vi "cRIO_8maze_controls_exo_wheelstart.vi"() -> ()   [LabVIEW 2019]
uses:
  <vilib>/Platform/TimedLoop/XDataNode/timing_clust.ctl
  <vilib>/Platform/TimedLoop/XDataNode/nitl_modes.ctl
  <vilib>/Platform/TimedLoop/XDataNode/wakeup.ctl
  Global 1.vi
  <vilib>/addons/control/pid/pid.llb/PID (DBL Array).vi
  <vilib>/imath/engines/lvmath2/RunTimeEngine/BuiltInFunctions/inv/NIMS_inv(GM).vi
  <instcachedir>/0/NIMS_inv(GM)_A6DF8FE880224208AACFE4CF9F659502.lvgen/NIMS_inv(GM)_A6DF8FE880224208AACFE4CF9F659502_000.vi
  <vilib>/imath/engines/lvmath2/RunTimeEngine/ArithmeticOperatorToken/NIMS_ArithmeticOperator_multmx(M,CV).vi
  <instcachedir>/0/NIMS_ArithmeticOperator_multmx(M,CV)_1D61EED49E1847F3B05DBB8EDD2FBF8F.lvgen/NIMS_ArithmeticOperator_multmx(M,CV)_1D61EED49E1847F3B05DBB8EDD2FBF8F_000.vi
  <vilib>/imath/engines/lvmath2/RunTimeEngine/ErrorHandling/NIMS_Create Error From Enums.vi
  <vilib>/imath/engines/lvmath2/RunTimeEngine/IndexRead/NIMS M(R2,S).vi
  <instcachedir>/0/NIMS M(R2,S)_56813DCFDD5A484292D2195AF15D2BF5.lvgen/NIMS M(R2,S)_56813DCFDD5A484292D2195AF15D2BF5_000.vi
  <vilib>/imathl/engines/lvmath/Functions/Error Handling/Create Error.vi
  <vilib>/imath/engines/lvmath2/RunTimeEngine/IndexRead/NIMS M(S,S).vi
  <instcachedir>/0/NIMS M(S,S)_AC51E74150A542F7991B9634C66F3096.lvgen/NIMS M(S,S)_AC51E74150A542F7991B9634C66F3096_000.vi
  <vilib>/imath/engines/lvmath2/RunTimeEngine/NodeEndStatement/NIMS_NodeEndStatement_Output.vi
  <instcachedir>/0/NIMS_NodeEndStatement_Output_53EC0D466D134D7ABD903AC30B43404B.lvgen/NIMS_NodeEndStatement_Output_53EC0D466D134D7ABD903AC30B43404B_001.vi
  <instcachedir>/0/NIMS_NodeEndStatement_Output_53EC0D466D134D7ABD903AC30B43404B.lvgen/NIMS_NodeEndStatement_Output_53EC0D466D134D7ABD903AC30B43404B_005.vi
  <vilib>/imath/engines/lvmath2/RunTimeEngine/ErrorHandling/NIMS_Finalize Error.vi
  <vilib>/platform/TimedLoop/XDataNode/XDataNode.xnode
  <vilib>/addons/control/pid/NI_PID_pid.lvlib
  <vilib>/Platform/TimedLoop/XDataNode/XDNodeRunTimeDep.lvlib
panel:
  in  "Reset sliders":bool=TRUE
  in  "MDServoPWM_R":dbl[](array[numeric])=[5.3, 8.5]
  in  "MDServoPWM_L":dbl[](array[numeric])=[4.6, 8.4]
  in  "Mouse off":bool
  in  "PWMset2":dbl[](array[numeric])=[8.1, 5.3, 8.5]
  in  "PWMset1":dbl[](array[numeric])=[3.4, 4.6, 8.2]
  in  "PWM positions":dbl[](array[numeric])=[8.7, 4.0, 4.4, 8.6]
  in  "PWM rate":dbl[](array[numeric])=[0.1, 0.1, 0.1, 0.1]
  out "appended array":bool[](array[boolean])
  in  "LED_L":bool
  in  "LED_R":bool
  in  "MD_L":bool
  in  "MD_R":bool
  out "Left":bool=TRUE
  in  "AIR":bool
  in  "Sound":bool
  out "Right":bool=TRUE
  in  "MD time (ms)":i32=3000
  in  "Loop seq.":dbl
  in  "Initialize":bool=TRUE
  in  "No Milk":bool
  out "All BBL":bool
  out "BB3_L":bool
  out "BB2_L":bool
  out "BB1_R":bool
  out "All BBR":bool
  out "BB3_R":bool
  out "BB2_R":bool
  out "BB1_L":bool
  out "Seq update":i32
  in  "Make sound":bool
  in  "Air puff time":u32=1000
  out "Direction array":bool[](array[boolean])=[TRUE, FALSE, FALSE, TRUE, FALSE, TRUE, TRUE, FALSE, TRUE, FALSE, FALSE, TRUE, FALSE, TRUE, FALSE, FALSE, TRUE, FALSE, TRUE, TRUE, FALSE, TRUE, FALSE, FALSE, TRUE, FALSE, TRUE, TRUE, FALSE, TRUE, FALSE, FALSE, TRUE, FALSE, TRUE, TRUE, FALSE, TRUE, FALSE, FALSE, TRUE, FALSE, TRUE, TRUE, FALSE, TRUE, FALSE, FALSE, TRUE]
  in  "manual homing stop":bool
  out "Homed":bool[](array[boolean])
  out "Hall voltages":dbl[](array[numeric])
  in  "Joint offset":dbl[](array[numeric])
  in  "Target HallV":dbl[](array[numeric])
  out "loop":i32
  in  "RETURN TO HOME \nPOSITION AND STOP":bool
  in  "lower limit":dbl[](array[numeric])=[-0.3, -0.36, -0.782, -6000.0]
  in  "upper limit":dbl[](array[numeric])=[0.3, 0.36, -0.65, 6000.0]
  in  "Yaw":dbl(slide) scale=0.0..3.142
  in  "Z":dbl(slide)=-0.7034810126582278 scale=-0.1..0.1
  in  "Y":dbl(slide) scale=-0.3..0.15
  in  "X":dbl(slide) scale=-0.15..0.15
  out "target position":dbl[](array[numeric])
  in  "Output range (PWM)":cluster{"output high":dbl, "output low":dbl}[](array[cluster])=[{"output high"=100.0, "output low"=-100.0}] {"output low" format="%.2f"; "output high" format="%.2f"}
  in  "Admittance PID gains":T1(array[cluster])=[{"proportional gain (Kc)"=1.0, "integral time (Ti, min)"=0.01, "derivative time (Td, min)"=0.0}] {"derivative time (Td, min)" format="%.3f"; "integral time (Ti, min)" format="%.3f"; "proportional gain (Kc)" format="%.3f"}
  in  "goniometer PWM\n offset":dbl=50.0
  in  "delta PWM offset":dbl[](array[numeric])=[50.0, 50.0, 50.0]
  in  "manual position\n(global frame)":dbl[](array[numeric])=[0.0, 0.0, 0.0, 0.0, 0.0, 0.0]
  in  "Out of range":bool
  out "True loop time (ms)":u32
  in  "theta6":dbl
  in  "theta1,2,3 pos2":dbl=-0.75
  in  "Initial pos 2":bool
  in  "Theta PID gains":T1(array[cluster])=[{"proportional gain (Kc)"=1.0, "integral time (Ti, min)"=0.01, "derivative time (Td, min)"=0.0}] {"derivative time (Td, min)" format="%.3f"; "integral time (Ti, min)" format="%.3f"; "proportional gain (Kc)" format="%.3f"}
  in  "Theta output range":cluster{"output high":dbl, "output low":dbl}[](array[cluster])=[{"output high"=100.0, "output low"=-100.0}] {"output low" format="%.2f"; "output high" format="%.2f"}
  in  "theta 6":dbl
  in  "theta1,2,3":dbl=-0.75
  in  "Stop Joint space control":bool
  in  "Disable PID":bool
  out "op-space pos\n(global frame)":dbl[](array[numeric])
  out "discriminant (>0)":dbl
  in  "Loop time (ms)":i64=10
  out "J":dbl[][](array[numeric])
  out "Joint_pos (rad)":dbl[](array[numeric])
  # "VALUE USED FOR INITIALISATION, TROUBLESHOOTING AND ANALYSIS"
  # "Initialise system; both buttons must be pressed sequentially, left then right. Press Stop JSC when AB offset = Joint_pos"
  # "STOP AND RETURN TO HOME"
  # "Use Manual position control to set up or adjust the headstage position; the sliders ADD ON to the current position."
  # "POSITION LIMITS"
  # "8 maze controls - air puff manually activated; 3000ms MD time = 8uL milk"
  # "NB: if True loop time does not equal Loop time\nthen the virtual admittance will not be correct"
  # "Trajectory parameters"
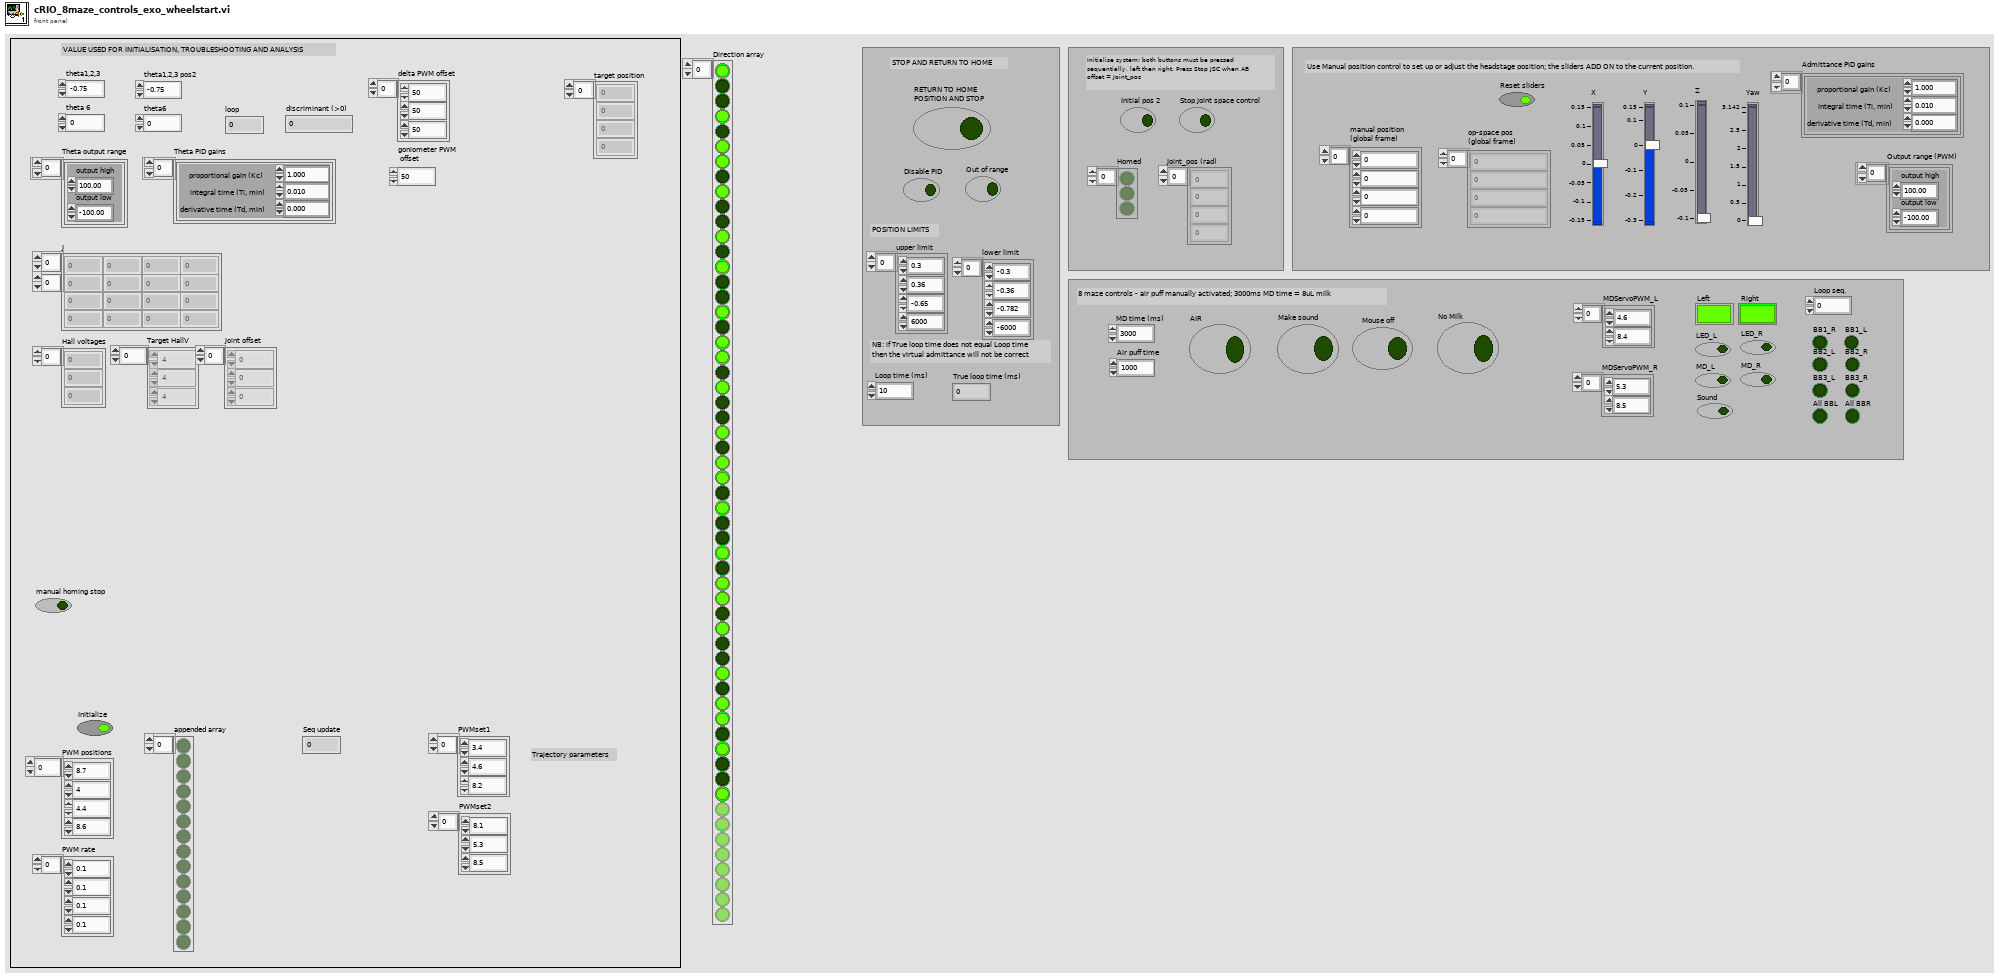
[diagram p1: front panel]
types:
  T1 = cluster{"proportional gain (Kc)":dbl, "integral time (Ti, min)":dbl, "derivative time (Td, min)":dbl}[]
  T2 = typedef "XDNodeRunTimeDep.lvlib/timing_clust.ctl" = cluster{"Expected End [f-1]":u64, "Actual End [f-1]":u64, "Finished Late? [f-1]":bool, "Expected End [i-1]":u64, "Actual End [i-1]":u64, "Finished Late? [i-1]":bool, "Expected Start [i]":u64, "Actual Start [i]":u64, "Expected Start [f]":u64, "Actual Start [f]":u64, "Source Name":string, "Structure Name":string, "Period":i64, "Deadline":i64, "Offset":i64, "Start":i64, "Priority":i32, "Timeout":i32, "Mode":T3, "Wakeup Reason":T4, "Error":errorcluster, "Source Type":string, "Secondary Source Type":string, "Global End Time":u64, "Global Start Time":u64, "Frame Duration":u64, "Iteration Duration":u64, "Assigned CPU":i32, "I/O Scan Engine Mode":u32}
  T3 = typedef "XDNodeRunTimeDep.lvlib/nitl_modes.ctl" = enum32{"No Change", "Process missed periods, maintain original phase", "Discard missed periods, maintain original phase", "Process missed periods, ignore original phase", "Discard missed periods, ignore original phase"}
  T4 = typedef "XDNodeRunTimeDep.lvlib/wakeup.ctl" = enum32{"Normal", "Aborted", "Asynchronous wakeup", "Timing source error", "Timed loop error", "Timeout"}
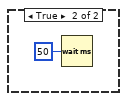
[diagram p2: hidden frame]
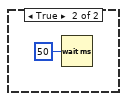
[diagram p3: hidden frame]
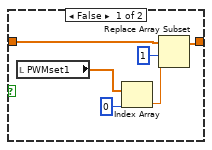
[diagram p5: hidden frame]
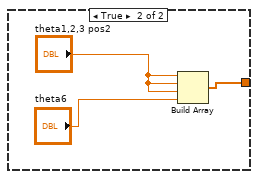
[diagram p6: hidden frame]
diagram:
  n1 = flat-sequence {
    frame #0 {
      w11 = 0.0 ("X")
      n2 = local write "RETURN TO HOME \nPOSITION AND STOP"(FALSE ("RETURN TO HOME \nPOSITION AND STOP")) -> ()
      n3 = local write "Initial pos 2"(FALSE ("Initial pos 2")) -> ()
      n4 = local write "Stop Joint space control"(FALSE ("Stop Joint space control")) -> ()
      n5 = local write "Disable PID"(TRUE ("Disable PID")) -> ()
      n6 = local write "Disable PID"(FALSE ("Enable PID")) -> ()
      n7 = local write "theta1,2,3 pos2"(-0.25 ("theta1,2,3 pos2")) -> ()
      n8 = local write "theta1,2,3"(-0.75 ("theta1,2,3")) -> ()
      n9 = global write "Global 1.vi" "a_1 (m)"(0.1 ("a_4 (m)")) -> ()
      n10 = local write "Yaw"(w11) -> ()
      n11 = local write "theta6"(0.0 ("theta4,5,6")) -> ()
      n12 = global write "Global 1.vi" "Rf (m)"(0.1898 ("Rf (m)")) -> ()
      n13 = global write "Global 1.vi" "Ld (m)"(0.656 ("Ld (m)")) -> ()
      n14 = global write "Global 1.vi" "L6 (m)"(0.22 ("a_4 (m)")) -> ()
      n15 = global write "Global 1.vi" "Rm (m)"(0.1 ("Rm (m)")) -> ()
      n16 = global write "Global 1.vi" "Lp (m)"(0.34 ("Lp (m)")) -> ()
      n17 = local write "Y"(w11) -> ()
      n18 = local write "X"(w11) -> ()
      n19 = local write "Z"(w11) -> ()
      n20 = local write "Theta output range"(cluster{"output high":dbl, "output low":dbl}[] [{"output high"=50.0, "output low"=-50.0}] ("XYZ output range")) -> ()
      n21 = local write "Theta PID gains"(T1 [{"proportional gain (Kc)"=10.0, "integral time (Ti, min)"=0.0, "derivative time (Td, min)"=0.0}] ("XYZ PID gains")) -> ()
      n22 = local write "Admittance PID gains"(T1 [{"proportional gain (Kc)"=80.0, "integral time (Ti, min)"=0.5, "derivative time (Td, min)"=0.0}, {"proportional gain (Kc)"=80.0, "integral time (Ti, min)"=0.5, "derivative time (Td, min)"=0.0}, {"proportional gain (Kc)"=40.0, "integral time (Ti, min)"=0.5, "derivative time (Td, min)"=0.0}, {"proportional gain (Kc)"=200.0, "integral time (Ti, min)"=0.0, "derivative time (Td, min)"=0.0}] ("XYZ PID gains")) -> ()
      n23 = local write "upper limit"(dbl[] [0.3, 0.36, -0.65, 6000.0] ("upper limit")) -> ()
      n24 = local write "Output range (PWM)"(cluster{"output high":dbl, "output low":dbl}[] [{"output high"=50.0, "output low"=-50.0}, {"output high"=50.0, "output low"=-50.0}, {"output high"=50.0, "output low"=-50.0}, {"output high"=50.0, "output low"=-50.0}] ("XYZ output range")) -> ()
      n25 = local write "lower limit"(dbl[] [-0.3, -0.36, -0.782, -6000.0] ("lower limit")) -> ()
      n26 = local write "Reset sliders"(FALSE ("Reset sliders")) -> ()
      n27 = local write "Target HallV"(dbl[] [1.0, 1.0, 1.0] ("Joint offset")) -> ()
    }
    frame #1 {
      n28 = while {
        stop <- w25 stop-if-true
        w37 = dbl[] [50.0, 50.0, 50.0]  # PWM 50% offset
        n29 = shared-variable "RT CompactRIO Target\\Mod8\\AI28"() -> (w45:dbl)  [unwired: 1 in, 1 out]
        n30 = shared-variable "RT CompactRIO Target\\Mod8\\AI27"() -> (w44:dbl)  [unwired: 1 in, 1 out]
        n31 = shared-variable "RT CompactRIO Target\\Mod8\\AI20"() -> (w46:dbl)  [unwired: 1 in, 1 out]
        n32 = Build Array(w46, w45, w44) -> (w33:dbl[])
        "Hall voltages" <- w33
        n33 = call-poly <vilib>:"PID.vi"("output range"=cluster{"output high":dbl, "output low":dbl}[] [{"output high"=5.0, "output low"=-5.0}], "PID gains"=T1 [{"proportional gain (Kc)"=1.0, "integral time (Ti, min)"=0.0, "derivative time (Td, min)"=0.0}], "process variable"=w33, "setpoint"="Target HallV") -> ("output"=w28:dbl[])  [unwired: 6 in, 1 out]
        n34 = Negate(x=w28) -> (-x=w27:dbl[])
        n35 = Add(x=w27, y=w37) -> (x+y=w36:dbl[])
        n36 = Add(x=dbl[] [0.3, 0.3, 0.3], y="Target HallV") -> (x+y=w32:dbl[])
        n37 = Index Array(array=w36, index=1) -> (element=w39:dbl)
        n38 = Index Array(array=w36, index=0) -> (element=w40:dbl)
        n39 = Index Array(array=w36, index=2) -> (element=w38:dbl)
        n40 = In Range and Coerce(upper limit=w32, x=w33, lower limit="Target HallV") -> (In Range?=w29:bool[])  [unwired: 1 out]
        "Homed" <- w29
        n41 = And Array Elements(Boolean array=w29) -> (logical AND=w26:bool)
        n42 = In Range and Coerce(upper limit=52.0, x=w40, lower limit=48.0) -> (coerced(x)=w49:dbl)  [unwired: 1 out]
        n43 = In Range and Coerce(upper limit=52.0, x=w39, lower limit=48.0) -> (coerced(x)=w48:dbl)  [unwired: 1 out]
        n44 = In Range and Coerce(upper limit=52.0, x=w38, lower limit=48.0) -> (coerced(x)=w47:dbl)  [unwired: 1 out]
        n45 = Or(x=w26, y="manual homing stop") -> (x .or. y?=w25:bool)
        n46 = shared-variable "RT CompactRIO Target\\Mod5\\PWM1"(w48) -> ()  [unwired: 1 in, 1 out]
        n47 = shared-variable "RT CompactRIO Target\\Mod5\\PWM2"(w47) -> ()  [unwired: 1 in, 1 out]
        n48 = shared-variable "RT CompactRIO Target\\Mod5\\PWM0"(w49) -> ()  [unwired: 1 in, 1 out]
      }
    }
    frame #2 {
      n49 = call "cRIO_4DoF_Encoders_counts2rad(subVI).vi"() -> ("Theta3"=w57:dbl, "Theta2"=w58:dbl, "Theta1"=w59:dbl, "Theta6"=w60:dbl)  [unwired: 4 in]
      n50 = Build Array(w59, w58, w57, w60) -> (w56:dbl[])
      n51 = local write "Joint offset"(w56) -> ()
    }
    frame #3 {
      n52 = while "Joint space control" {
        stop <- w68 stop-if-true
        w71 = dbl[] [50.0, 50.0, 50.0, 50.0]  # PWM 50% offset
        n53 = case shown="False" "Initial pos 2" {
          tunnel: [w93 w94] -> w88
          frame False {
            n54 = Build Array("theta1,2,3", "theta1,2,3", "theta1,2,3", "theta 6") -> (w93:dbl[])
          }
          frame True {
            n55 = Build Array("theta1,2,3 pos2", "theta1,2,3 pos2", "theta1,2,3 pos2", "theta6") -> (w94:dbl[])
          }
        }
        n56 = local read "Joint_pos (rad)"() -> (w62:dbl[])
        n57 = call-poly <vilib>:"PID.vi"("output range"="Theta output range", "PID gains"="Theta PID gains", "process variable"=w62, "setpoint"=w88) -> ("output"=w61:dbl[])  [unwired: 6 in, 1 out]
        n58 = Add(x=w61, y=w71) -> (x+y=w70:dbl[])
        n59 = Index Array(array=w70, index=0) -> (element=w83:dbl)
        n60 = Index Array(array=w70, index=1) -> (element=w74:dbl)
        n61 = Index Array(array=w70, index=2) -> (element=w73:dbl)
        n62 = Index Array(array=w70, index=3) -> (element=w72:dbl)
        n63 = In Range and Coerce(upper limit=99.0, x=w83, lower limit=1.0) -> (coerced(x)=w66:dbl)  [unwired: 1 out]
        n64 = In Range and Coerce(upper limit=99.0, x=w74, lower limit=1.0) -> (coerced(x)=w65:dbl)  [unwired: 1 out]
        n65 = In Range and Coerce(upper limit=99.0, x=w72, lower limit=1.0) -> (coerced(x)=w63:dbl)  [unwired: 1 out]
        n66 = In Range and Coerce(upper limit=99.0, x=w73, lower limit=1.0) -> (coerced(x)=w64:dbl)  [unwired: 1 out]
        n67 = shared-variable "RT CompactRIO Target\\Mod5\\PWM2"(w64) -> ()  [unwired: 1 in, 1 out]
        n68 = shared-variable "RT CompactRIO Target\\Mod5\\PWM3"(w63) -> ()  [unwired: 1 in, 1 out]
        n69 = shared-variable "RT CompactRIO Target\\Mod5\\PWM0"(w66) -> ()  [unwired: 1 in, 1 out]
        n70 = shared-variable "RT CompactRIO Target\\Mod5\\PWM1"(w65) -> ()  [unwired: 1 in, 1 out]
        n71 = And(x="Stop Joint space control", y="Initial pos 2") -> (x .and. y?=w68:bool)
      }
    }
    frame #4 {
      w113 = dbl[] [50.0, 50.0, 50.0, 50.0] ("y")
      w119 = 0.0 ("X")
      n72 = Wait (ms)(milliseconds to wait=u32 50) -> ()  [unwired: 1 out]
      n73 = Index Array(array=w113, index=0) -> (element=w100:dbl)
      n74 = Index Array(array=w113, index=1) -> (element=w99:dbl)
      n75 = Index Array(array=w113, index=2) -> (element=w98:dbl)
      n76 = Index Array(array=w113, index=3) -> (element=w97:dbl)
      n77 = local write "Yaw"(w119) -> ()
      n78 = local write "Z"(w119) -> ()
      n79 = local write "Y"(w119) -> ()
      n80 = In Range and Coerce(upper limit=99.0, x=w100, lower limit=1.0) -> (coerced(x)=w104:dbl)  [unwired: 1 out]
      n81 = local write "X"(w119) -> ()
      n82 = In Range and Coerce(upper limit=99.0, x=w99, lower limit=1.0) -> (coerced(x)=w103:dbl)  [unwired: 1 out]
      n83 = In Range and Coerce(upper limit=99.0, x=w98, lower limit=1.0) -> (coerced(x)=w102:dbl)  [unwired: 1 out]
      n84 = In Range and Coerce(upper limit=99.0, x=w97, lower limit=1.0) -> (coerced(x)=w101:dbl)  [unwired: 1 out]
      n85 = shared-variable "RT CompactRIO Target\\Mod5\\PWM0"(w104) -> ()  [unwired: 1 in, 1 out]
      n86 = shared-variable "RT CompactRIO Target\\Mod5\\PWM1"(w103) -> ()  [unwired: 1 in, 1 out]
      n87 = shared-variable "RT CompactRIO Target\\Mod5\\PWM2"(w102) -> ()  [unwired: 1 in, 1 out]
      n88 = shared-variable "RT CompactRIO Target\\Mod5\\PWM3"(w101) -> ()  [unwired: 1 in, 1 out]
    }
    frame #5 {
      n89 = node-c288("Loop time (ms)") -> (w122:T2)  [unwired: 3 in]
      n90 = timed-loop {
        shift-right: [w187] -> _
        shift-left: _ -> [w186]
        timing: w122 -> [_]
        timing-out: [_] -> w121
        i -> [w168]
        stop <- "RETURN TO HOME \nPOSITION AND STOP" stop-if-true
        n91 = node-c288() -> ()  [unwired: 1 in, 1 out]
        n92 = local read "Joint_pos (rad)"() -> (w154:dbl[])
        n93 = Build Array("X", "Y", "Z", "Yaw") -> (w146:dbl[])
        n94 = Index Array(array=w154, index=0) -> (element=w156:dbl)
        n95 = Index Array(array=w154, index=1) -> (element=w155:dbl)
        n96 = Index Array(array=w154, index=2) -> (element=w153:dbl)
        n97 = Index Array(array=w154, index=3) -> (element=w152:dbl)
        n98 = Less?(x=w168, y=10) -> (x < y?=w124:bool)
        n99 = Add(x="manual position\n(global frame)", y=w146) -> (x+y=w126:dbl[])
        n100 = call "cRIO_4DoF_Delta_forward_kinematics.vi"("theta3"=w153, "theta2"=w155, "theta1"=w156) -> ("YD"=w159:cdb, "ZD"=w160:cdb, "discriminant (>0)"=→"discriminant (>0)":dbl, "XD"=w158:cdb)  [unwired: 5 in]
        n101 = Or(x="Reset sliders", y=w124) -> (x .or. y?=w125:bool)
        n102 = case shown="True" w125 {
          tunnel: [w196 w199] -> w145
          tunnel: w126 -> [w196 _]
          frame False {
          }
          frame True {
            w198 = 0.0 ("Z")
            n103 = local read "op-space pos\n(global frame)"() -> (w199:dbl[])
            n104 = local write "manual position\n(global frame)"(w199) -> ()
            n105 = local write "target position"(w199) -> ()
            n106 = local write "Yaw"(w198) -> ()
            n107 = local write "X"(w198) -> ()
            n108 = local write "Y"(w198) -> ()
            n109 = local write "Z"(w198) -> ()
            n110 = local write "Reset sliders"(FALSE ("Reset sliders")) -> ()
          }
        }
        n111 = call "cRIO_4DoF_Gonio_forward_kinematics.vi"("X in"=w158, "Y in"=w159, "Z in"=w160, "Theta6_meas"=w152) -> ("X out"=w166:dbl, "Y out"=w165:dbl, "Z out"=w164:dbl, "yaw"=w163:dbl)  [unwired: 7 in, 1 out]
        n112 = call "cRIO_4DOF_Jacobian_v3.vi"("XD"=w158, "YD"=w159, "ZD"=w160, "Joint positions"=w154) -> ("J"=→"J":dbl[][])  [unwired: 7 in]
        n113 = Build Array(w166, w165, w164, w163) -> (→"op-space pos\n(global frame)":dbl[])
        n114 = local read "op-space pos\n(global frame)"() -> (w178:dbl[])
        n115 = In Range and Coerce(upper limit="upper limit", x=w145, lower limit="lower limit") -> (coerced(x)=w144:dbl[])  [unwired: 1 out]
        "target position" <- w144
        n116 = call-poly <vilib>:"PID.vi"("output range"="Output range (PWM)", "PID gains"="Admittance PID gains", "process variable"=w178, "setpoint"=w144) -> ("output"=w127:dbl[])  [unwired: 6 in, 1 out]
        n117 = local read "J"() -> (w175:dbl[][])
        n118 = mathscript code="opspace = [op_vel]';\njointspace = inv(J)*opspace;\nlinrad = real(jointspace(1:3,1));\nrotrad = real(jointspace(4,1));" "Velocity conversion (in PWM space)"("op_vel"=w127, "J"=w175) -> ("linrad"=w189:dbl[], "rotrad"=w192:dbl)  [unwired: 1 in, 1 out]
        n119 = Compound Arithmetic op=OR(w124, "Disable PID", "Out of range") -> (w183:bool)
        n120 = Add(x=w189, y="delta PWM offset") -> (x+y=w191:dbl[])
        n121 = Add(x=w192, y="goniometer PWM\n offset") -> (x+y=w190:dbl)
        n122 = case shown="False" w183 {
          tunnel: w191 -> [w296 _]
          tunnel: w190 -> [w295 _]
          tunnel: [w296 w297] -> w179
          tunnel: [w295 w298] -> w128
          tunnel: "goniometer PWM\n offset" -> [_ w298]
          tunnel: "delta PWM offset" -> [_ w297]
          frame False {
          }
          frame True {
          }
        }
        n123 = Index Array(array=w179, index=1) -> (element=w130:dbl)
        n124 = Index Array(array=w179, index=2) -> (element=w129:dbl)
        n125 = Index Array(array=w179, index=0) -> (element=w131:dbl)
        n126 = Tick Count (ms)() -> (millisecond timer value=w187:u32)
        n127 = In Range and Coerce(upper limit=99.0, x=w131, lower limit=1.0) -> (coerced(x)=w135:dbl)  [unwired: 1 out]
        n128 = In Range and Coerce(upper limit=99.0, x=w130, lower limit=1.0) -> (coerced(x)=w134:dbl)  [unwired: 1 out]
        n129 = In Range and Coerce(upper limit=99.0, x=w129, lower limit=1.0) -> (coerced(x)=w133:dbl)  [unwired: 1 out]
        n130 = In Range and Coerce(upper limit=99.0, x=w128, lower limit=1.0) -> (coerced(x)=w132:dbl)  [unwired: 1 out]
        n131 = Subtract(x=w187, y=w186) -> (x-y=→"True loop time (ms)":u32)
        n132 = shared-variable "RT CompactRIO Target\\Mod5\\PWM2"(w133) -> ()  [unwired: 1 in, 1 out]
        n133 = shared-variable "RT CompactRIO Target\\Mod5\\PWM0"(w135) -> ()  [unwired: 1 in, 1 out]
        n134 = shared-variable "RT CompactRIO Target\\Mod5\\PWM1"(w134) -> ()  [unwired: 1 in, 1 out]
        n135 = shared-variable "RT CompactRIO Target\\Mod5\\PWM3"(w132) -> ()  [unwired: 1 in, 1 out]
        n136 = node-c288() -> ()  [unwired: 1 in, 1 out]
        "loop" <- w168
      }
      n137 = node-c288(w121) -> ()  [unwired: 1 out]
    }
    frame #6 {
      n138 = while "Joint space control" {
        stop <- FALSE stop-if-true
        n139 = local read "Joint_pos (rad)"() -> (w319:dbl[])
        n140 = local read "theta1,2,3"() -> (w324:dbl)
        n141 = local read "theta6"() -> (w323:dbl)
        n142 = Build Array(w324, w324, w324, w323) -> (w332:dbl[])
        n143 = local read "Theta output range"() -> (w320:cluster{"output high":dbl, "output low":dbl}[])
        n144 = local read "Theta PID gains"() -> (w321:T1)
        n145 = call-poly <vilib>:"PID.vi"("output range"=w320, "PID gains"=w321, "process variable"=w319, "setpoint"=w332) -> ("output"=w327:dbl[])  [unwired: 6 in, 1 out]
        n146 = Add(x=w327, y=dbl[] [50.0, 50.0, 50.0, 50.0]) -> (x+y=w325:dbl[])
        n147 = Index Array(array=w325, index=0) -> (element=w306:dbl)
        n148 = Index Array(array=w325, index=1) -> (element=w305:dbl)
        n149 = Index Array(array=w325, index=2) -> (element=w304:dbl)
        n150 = Index Array(array=w325, index=3) -> (element=w303:dbl)
        n151 = In Range and Coerce(upper limit=99.0, x=w306, lower limit=1.0) -> (coerced(x)=w310:dbl)  [unwired: 1 out]
        n152 = In Range and Coerce(upper limit=99.0, x=w305, lower limit=1.0) -> (coerced(x)=w309:dbl)  [unwired: 1 out]
        n153 = In Range and Coerce(upper limit=99.0, x=w304, lower limit=1.0) -> (coerced(x)=w308:dbl)  [unwired: 1 out]
        n154 = In Range and Coerce(upper limit=99.0, x=w303, lower limit=1.0) -> (coerced(x)=w307:dbl)  [unwired: 1 out]
        n155 = shared-variable "RT CompactRIO Target\\Mod5\\PWM0"(w310) -> ()  [unwired: 1 in, 1 out]
        n156 = shared-variable "RT CompactRIO Target\\Mod5\\PWM2"(w308) -> ()  [unwired: 1 in, 1 out]
        n157 = shared-variable "RT CompactRIO Target\\Mod5\\PWM1"(w309) -> ()  [unwired: 1 in, 1 out]
        n158 = shared-variable "RT CompactRIO Target\\Mod5\\PWM3"(w307) -> ()  [unwired: 1 in, 1 out]
      }
    }
  }
  n159 = while "Avoid Delta robot joint collision with platform" {
    stop <- FALSE stop-if-true
    n160 = local read "Joint_pos (rad)"() -> (w339:dbl[])
    n161 = Wait (ms)(milliseconds to wait=u32 25) -> ()  [unwired: 1 out]
    n162 = Array Subset(array=w339, index=0, length=3) -> (w336:dbl[])
    n163 = Less?(x=w336, y=dbl[] [-0.85, -0.85, -0.85]) -> (x < y?=w341:bool[])
    n164 = Or Array Elements(Boolean array=w341) -> (logical OR=w333:bool)
    n165 = local write "Out of range"(w333) -> ()
  }
  n166 = while "Encoder counts to Joint position" {
    stop <- FALSE stop-if-true
    n167 = local read "Loop time (ms)"() -> (w354:i64)
    n168 = call "cRIO_4DoF_Encoders_counts2rad(subVI).vi"() -> ("Theta3"=w349:dbl, "Theta2"=w350:dbl, "Theta1"=w351:dbl, "Theta6"=w355:dbl)  [unwired: 4 in]
    n169 = Build Array(w351, w350, w349, w355) -> (w348:dbl[])
    n170 = Divide "offset"(x=3.141592653589793, y=4.0) -> (x/y=w347:dbl)
    n171 = Wait (ms)(milliseconds to wait=w354) -> ()  [unwired: 1 out]
    n172 = Build Array(w347, w347, w347, 0.0 ("element")) -> (w345:dbl[])
    n173 = Subtract(x=w348, y=w345) -> (x-y=w344:dbl[])
    n174 = Subtract(x=w344, y="Joint offset") -> (x-y=→"Joint_pos (rad)":dbl[])
  }
  n175 = while {
    stop <- FALSE stop-if-true
    n176 = Wait (ms)(milliseconds to wait=u32 250) -> ()  [unwired: 1 out]
    n177 = shared-variable "RT CompactRIO Target\\Mod1\\DI2"() -> (w360:bool)  [unwired: 1 in, 1 out]
    n178 = shared-variable "RT CompactRIO Target\\Mod1\\DI3"() -> (w359:bool)  [unwired: 1 in, 1 out]
    n179 = shared-variable "RT CompactRIO Target\\Mod1\\DI0"() -> (w362:bool)  [unwired: 1 in, 1 out]
    n180 = shared-variable "RT CompactRIO Target\\Mod1\\DI1"() -> (w361:bool)  [unwired: 1 in, 1 out]
    n181 = Not(x=w360) -> (.not. x?=w364:bool)
    n182 = Not(x=w359) -> (.not. x?=w363:bool)
    n183 = Not(x=w362) -> (.not. x?=w366:bool)
    n184 = Not(x=w361) -> (.not. x?=w365:bool)
    n185 = shared-variable "RT CompactRIO Target\\Mod6\\DIO2"(w364) -> ()  [unwired: 1 in, 1 out]
    n186 = shared-variable "RT CompactRIO Target\\Mod6\\DIO3"(w363) -> ()  [unwired: 1 in, 1 out]
    n187 = shared-variable "RT CompactRIO Target\\Mod1\\DO2"(w360) -> ()  [unwired: 1 in, 1 out]
    n188 = shared-variable "RT CompactRIO Target\\Mod1\\DO3"(w359) -> ()  [unwired: 1 in, 1 out]
    n189 = shared-variable "RT CompactRIO Target\\Mod6\\DIO0"(w366) -> ()  [unwired: 1 in, 1 out]
    n190 = shared-variable "RT CompactRIO Target\\Mod6\\DIO1"(w365) -> ()  [unwired: 1 in, 1 out]
    n191 = shared-variable "RT CompactRIO Target\\Mod1\\DO0"(w362) -> ()  [unwired: 1 in, 1 out]
    n192 = shared-variable "RT CompactRIO Target\\Mod1\\DO1"(w361) -> ()  [unwired: 1 in, 1 out]
  }
  n193 = flat-sequence {
    frame #0 {
      w368 = FALSE
      w371 = FALSE
      w372 = bool[] [TRUE, FALSE, TRUE, FALSE, TRUE, FALSE, TRUE, FALSE, TRUE, FALSE, TRUE, FALSE, TRUE, FALSE, TRUE, FALSE, TRUE, FALSE, TRUE, FALSE, TRUE, FALSE, TRUE, FALSE, TRUE, FALSE, TRUE, FALSE, TRUE, FALSE, TRUE, FALSE, TRUE, FALSE, TRUE, FALSE, TRUE, FALSE, TRUE, FALSE, TRUE, FALSE, TRUE, FALSE, TRUE, FALSE, TRUE, FALSE, TRUE, FALSE, TRUE, FALSE, TRUE, FALSE, TRUE, FALSE, TRUE, FALSE, TRUE, FALSE, TRUE, FALSE, TRUE, FALSE, TRUE, FALSE, TRUE, FALSE, TRUE, FALSE, TRUE]  # Alternating
      (unwired) bool[] [TRUE, FALSE, FALSE, TRUE, FALSE, TRUE, TRUE, FALSE, TRUE, FALSE, FALSE, TRUE, FALSE, TRUE, FALSE, FALSE, TRUE, FALSE, TRUE, TRUE, FALSE, TRUE, FALSE, FALSE, TRUE, FALSE, TRUE, TRUE, FALSE, TRUE, FALSE, FALSE, TRUE, FALSE, TRUE, TRUE, FALSE, TRUE, FALSE, FALSE, TRUE, FALSE, TRUE, TRUE, FALSE, TRUE, FALSE, FALSE, TRUE, FALSE, TRUE, TRUE, FALSE, TRUE, FALSE, FALSE, TRUE, FALSE, TRUE, TRUE, FALSE, TRUE, FALSE, FALSE, TRUE, FALSE, TRUE, TRUE, FALSE, TRUE, FALSE]  # Psuedo random
      w370 = TRUE
      w369 = FALSE
      n194 = local write "All BBR"(w371) -> ()
      n195 = local write "All BBL"(w371) -> ()
      n196 = local write "BB3_R"(w371) -> ()
      n197 = local write "BB1_R"(w371) -> ()
      n198 = local write "BB3_L"(w371) -> ()
      n199 = local write "BB1_L"(w371) -> ()
      n200 = local write "BB2_R"(w371) -> ()
      n201 = local write "BB2_L"(w371) -> ()
      n202 = local write "Initialize"(w370) -> ()
      n203 = local write "Sound"(w370) -> ()
      n204 = local write "No Milk"(w369) -> ()
      n205 = shared-variable "RT CompactRIO Target\\Mod6\\DIO29"(w369) -> ()  [unwired: 1 in, 1 out]
      n206 = shared-variable "RT CompactRIO Target\\Mod6\\DIO14"(w369) -> ()  [unwired: 1 in, 1 out]
      n207 = shared-variable "RT CompactRIO Target\\Mod6\\DIO20"(w369) -> ()  [unwired: 1 in, 1 out]
      n208 = shared-variable "RT CompactRIO Target\\Mod6\\DIO30"(w369) -> ()  [unwired: 1 in, 1 out]
      n209 = shared-variable "RT CompactRIO Target\\Mod6\\DIO7"(w369) -> ()  [unwired: 1 in, 1 out]
      n210 = shared-variable "RT CompactRIO Target\\Mod6\\DIO20"(w369) -> ()  [unwired: 1 in, 1 out]
      n211 = shared-variable "RT CompactRIO Target\\Mod6\\DIO17"(w370) -> ()  [unwired: 1 in, 1 out]
      n212 = local write "Loop seq."(0.0 ("Loop seq.")) -> ()
      n213 = local write "PWM positions"(dbl[] [9.5, 8.1, 4.4, 8.6]) -> ()
      n214 = local write "LED_L"(TRUE ("LED_L")) -> ()
      n215 = local write "LED_R"(w368) -> ()
      n216 = local write "Mouse off"(w368) -> ()
      "Direction array" <- w372
    }
    frame #1 {
      n217 = while "Loop sequence Right" {
        stop <- FALSE stop-if-true
        n218 = flat-sequence {
          frame #0 {
            # "Check sequence for right turn"
            n219 = while {
              stop <- w437 stop-if-true
              n220 = local read "Right"() -> (w437:bool)
              n221 = Wait (ms)(milliseconds to wait=u32 10) -> ()  [unwired: 1 out]
            }
          }
          frame #1 {
            # "Breakbeam 1 Left"
            n222 = while {
              shift-right: [w440] -> _
              shift-left: FALSE -> [w444]
              stop <- w439 stop-if-true
              n223 = shared-variable "RT CompactRIO Target\\Mod6\\DIO15"() -> (w440:bool)  [unwired: 1 in, 1 out]
              n224 = Wait (ms)(milliseconds to wait=u32 10) -> ()  [unwired: 1 out]
              n225 = local read "Initialize"() -> (w441:bool)
              n226 = Less?(x=w440, y=w444) -> (x < y?=w442:bool)
              n227 = Or(x=w442, y=w441) -> (x .or. y?=w439:bool)
              "BB1_L" <- w439
            }
          }
          frame #2 {
            # "Breakbeam 2 Right"
            n228 = while {
              stop <- w446 stop-if-true
              w446 = TRUE ("BB2_R")
              n229 = Wait (ms)(milliseconds to wait=u32 10) -> ()  [unwired: 1 out]
              "BB2_R" <- w446
            }
            n230 = local write "Initialize"(FALSE ("Initialize")) -> ()
          }
          frame #3 {
            # "Breakbeam 3 Right"
            n231 = while {
              shift-right: [w449] -> _
              shift-left: _ -> [w451]
              stop <- w448 stop-if-true
              n232 = shared-variable "RT CompactRIO Target\\Mod6\\DIO13"() -> (w449:bool)  [unwired: 1 in, 1 out]
              n233 = Wait (ms)(milliseconds to wait=u32 10) -> ()  [unwired: 1 out]
              n234 = Less?(x=w449, y=w451) -> (x < y?=w448:bool)
              "BB3_R" <- w448
            }
          }
          frame #4 {
            # "Servo 1 position"
            n235 = local read "PWM positions"() -> (w458:dbl[])
            n236 = Wait (ms)(milliseconds to wait=u32 50) -> ()  [unwired: 1 out]
            n237 = Replace Array Subset(array=w458, new element=8.7 ("new element/subarray"), index=0) -> (w453:dbl[])
            n238 = Replace Array Subset(array=w453, new element="MDServoPWM_R", index=2) -> (w452:dbl[])
            n239 = local write "PWM positions"(w452) -> ()
            "All BBR" <- TRUE
          }
          frame #5 {
            # "Wait for mouse to reach MD stop point"
            n240 = Wait (ms)(milliseconds to wait=u32 100) -> ()  [unwired: 1 out]
          }
          frame #6 {
            w463 = FALSE
            # "Disable X and reset indicators"
            n241 = local write "All BBR"(w463) -> ()
            n242 = local write "BB1_R"(w463) -> ()
            n243 = local write "BB1_L"(w463) -> ()
            n244 = local write "BB2_R"(w463) -> ()
            n245 = local write "BB3_R"(w463) -> ()
            n246 = Wait (ms)(milliseconds to wait=u32 100) -> ()  [unwired: 1 out]
          }
          frame #7 {
            n247 = Wait (ms)(milliseconds to wait=u32 100) -> ()  [unwired: 1 out]
          }
          frame #8 {
            n248 = local write "MD_R"(TRUE ("MD_R")) -> ()
            n249 = local write "LED_L"(TRUE ("LED_L")) -> ()
            n250 = local write "LED_R"(FALSE ("LED_R")) -> ()
            n251 = Wait (ms)(milliseconds to wait=u32 100) -> ()  [unwired: 1 out]
          }
        }
      }
      n252 = while "Loop sequence Left" {
        stop <- FALSE stop-if-true
        n253 = flat-sequence {
          frame #0 {
            # "Check sequence for left turn"
            n254 = while {
              stop <- w488 stop-if-true
              n255 = local read "Left"() -> (w488:bool)
              n256 = Wait (ms)(milliseconds to wait=u32 10) -> ()  [unwired: 1 out]
            }
          }
          frame #1 {
            # "Breakbeam 1 Right"
            n257 = while {
              shift-right: [w490] -> _
              shift-left: FALSE -> [w495]
              stop <- w491 stop-if-true
              n258 = shared-variable "RT CompactRIO Target\\Mod6\\DIO31"() -> (w490:bool)  [unwired: 1 in, 1 out]
              n259 = Wait (ms)(milliseconds to wait=u32 10) -> ()  [unwired: 1 out]
              n260 = local read "Initialize"() -> (w492:bool)
              n261 = Less?(x=w490, y=w495) -> (x < y?=w493:bool)
              n262 = Or(x=w493, y=w492) -> (x .or. y?=w491:bool)
              "BB1_R" <- w491
            }
          }
          frame #2 {
            # "Breakbeam 2 Left"
            n263 = while {
              stop <- w497 stop-if-true
              w497 = TRUE ("BB2_L")
              n264 = Wait (ms)(milliseconds to wait=u32 10) -> ()  [unwired: 1 out]
              "BB2_L" <- w497
            }
            n265 = local write "Initialize"(FALSE ("Initialize")) -> ()
          }
          frame #3 {
            # "Breakbeam 3 Left"
            n266 = while {
              shift-right: [w500] -> _
              shift-left: _ -> [w502]
              stop <- w499 stop-if-true
              n267 = shared-variable "RT CompactRIO Target\\Mod6\\DIO21"() -> (w500:bool)  [unwired: 1 in, 1 out]
              n268 = Wait (ms)(milliseconds to wait=u32 10) -> ()  [unwired: 1 out]
              n269 = Less?(x=w500, y=w502) -> (x < y?=w499:bool)
              "BB3_L" <- w499
            }
          }
          frame #4 {
            # "Servo 1 position"
            n270 = local read "PWM positions"() -> (w509:dbl[])
            n271 = Wait (ms)(milliseconds to wait=u32 50) -> ()  [unwired: 1 out]
            n272 = Replace Array Subset(array=w509, new element=4.5 ("new element/subarray"), index=0) -> (w504:dbl[])
            n273 = Replace Array Subset(array=w504, new element="MDServoPWM_L", index=2) -> (w503:dbl[])
            n274 = local write "PWM positions"(w503) -> ()
            "All BBL" <- TRUE
          }
          frame #5 {
            # "Wait for mouse to reach MD stop point"
            n275 = Wait (ms)(milliseconds to wait=u32 100) -> ()  [unwired: 1 out]
          }
          frame #6 {
            w513 = FALSE
            # "Reset indicators"
            n276 = Wait (ms)(milliseconds to wait=u32 100) -> ()  [unwired: 1 out]
            n277 = local write "All BBL"(w513) -> ()
            n278 = local write "BB1_L"(w513) -> ()
            n279 = local write "BB1_R"(w513) -> ()
            n280 = local write "BB2_L"(w513) -> ()
            n281 = local write "BB3_L"(w513) -> ()
          }
          frame #7 {
            n282 = Wait (ms)(milliseconds to wait=u32 100) -> ()  [unwired: 1 out]
          }
          frame #8 {
            n283 = local write "LED_L"(FALSE ("LED_L")) -> ()
            n284 = local write "LED_R"(TRUE ("LED_R")) -> ()
            n285 = Wait (ms)(milliseconds to wait=u32 100) -> ()  [unwired: 1 out]
            n286 = local write "MD_L"(TRUE ("MD_L")) -> ()
          }
        }
      }
      n287 = while "Control outputs, Inputs, and Left/Right switch" {
        stop <- FALSE stop-if-true
        w540 = dbl[] [8.7, 8.1, 4.4, 8.6]
        n288 = shared-variable "RT CompactRIO Target\\Mod6\\DIO15"() -> (w534:bool)  [unwired: 1 in, 1 out]
        n289 = shared-variable "RT CompactRIO Target\\Mod6\\DIO31"() -> (w528:bool)  [unwired: 1 in, 1 out]
        n290 = shared-variable "RT CompactRIO Target\\Mod6\\DIO21"() -> (w529:bool)  [unwired: 1 in, 1 out]
        n291 = shared-variable "RT CompactRIO Target\\Mod6\\DIO28"() -> (w531:bool)  [unwired: 1 in, 1 out]
        n292 = shared-variable "RT CompactRIO Target\\Mod6\\DIO13"() -> (w532:bool)  [unwired: 1 in, 1 out]
        n293 = shared-variable "RT CompactRIO Target\\Mod6\\DIO5"() -> (w530:bool)  [unwired: 1 in, 1 out]
        n294 = Build Array(w534, w528, w529, w530, w531, w532) -> (→"appended array":bool[])
        n295 = feedback #1(w540) -> (w541:dbl[])
        n296 = feedback #2(w540) -> (w544:dbl[])
        n297 = local read "Direction array"() -> (w521:bool[])
        n298 = In Range and Coerce(upper limit=w544, x="PWM positions", lower limit=w541) -> (coerced(x)=w543:dbl[])  [unwired: 1 out]
        n299 = Subtract(x=w543, y="PWM rate") -> (x-y=w542:dbl[])
        n300 = Add(x=w543, y="PWM rate") -> (x+y=w545:dbl[])
        n301 = feedback-in #1(w542) -> ()
        n302 = feedback-in #2(w545) -> ()
        n303 = Index Array(array=w543, index=0) -> (element=w524:dbl)
        n304 = Index Array(array=w543, index=1) -> (element=w523:dbl)
        n305 = Index Array(array=w543, index=2) -> (element=w553:dbl)
        n306 = Index Array(array=w543, index=3) -> (element=w554:dbl)
        n307 = Index Array(array=w521, index="Loop seq.") -> (element=w522:bool)
        "Left" <- w522
        n308 = shared-variable "RT CompactRIO Target\\Mod5\\PWM7"(w524) -> ()  [unwired: 1 in, 1 out]
        n309 = shared-variable "RT CompactRIO Target\\Mod5\\PWM4"(w523) -> ()  [unwired: 1 in, 1 out]
        n310 = shared-variable "RT CompactRIO Target\\Mod5\\PWM5"(w553) -> ()  [unwired: 1 in, 1 out]
        n311 = shared-variable "RT CompactRIO Target\\Mod5\\PWM6"(w554) -> ()  [unwired: 1 in, 1 out]
        n312 = Not(x=w522) -> (.not. x?=→"Right":bool)
        n313 = Wait (ms)(milliseconds to wait=u32 5) -> ()  [unwired: 1 out]
        n314 = shared-variable "RT CompactRIO Target\\Mod6\\DIO20"("LED_L") -> ()  [unwired: 1 in, 1 out]
        n315 = shared-variable "RT CompactRIO Target\\Mod6\\DIO29"("MD_L") -> ()  [unwired: 1 in, 1 out]
        n316 = shared-variable "RT CompactRIO Target\\Mod6\\DIO14"("MD_R") -> ()  [unwired: 1 in, 1 out]
        n317 = shared-variable "RT CompactRIO Target\\Mod6\\DIO30"("LED_R") -> ()  [unwired: 1 in, 1 out]
        n318 = shared-variable "RT CompactRIO Target\\Mod6\\DIO6"("AIR") -> ()  [unwired: 1 in, 1 out]
        n319 = shared-variable "RT CompactRIO Target\\Mod6\\DIO17"("Sound") -> ()  [unwired: 1 in, 1 out]
      }
      n320 = while {
        i -> [w418]
        stop <- FALSE stop-if-true
        n321 = flat-sequence {
          frame #0 {
            n322 = while {
              stop <- w421 stop-if-true
              n323 = local read "All BBR"() -> (w422:bool)
              n324 = local read "All BBL"() -> (w423:bool)
              n325 = Or(x=w423, y=w422) -> (x .or. y?=w421:bool)
              n326 = Wait (ms)(milliseconds to wait=u32 100) -> ()  [unwired: 1 out]
            }
          }
          frame #1 {
            n327 = for {
              N: 1 -> [_]
              n328 = local read "Loop seq."() -> (w428:dbl)
              n329 = Add(x=w428, y=1.0) -> (x+y=w426:dbl)
              n330 = local write "Loop seq."(w426) -> ()
            }
          }
          frame #2 {
            n331 = while {
              stop <- w429 stop-if-true
              n332 = local read "All BBR"() -> (w432:bool)
              n333 = local read "All BBL"() -> (w433:bool)
              n334 = Not(x=w432) -> (.not. x?=w430:bool)
              n335 = Not(x=w433) -> (.not. x?=w431:bool)
              n336 = Wait (ms)(milliseconds to wait=u32 100) -> ()  [unwired: 1 out]
              n337 = And(x=w431, y=w430) -> (x .and. y?=w429:bool)
            }
          }
        }
        n338 = Wait (ms)(milliseconds to wait=u32 100) -> ()  [unwired: 1 out]
        "Seq update" <- w418
      }
      n339 = while "Sound timing" {
        stop <- FALSE stop-if-true
        n340 = Wait (ms)(milliseconds to wait=u32 50) -> ()  [unwired: 1 out]
        n341 = case shown="True" "Make sound" {
          frame False {
          }
          frame True {
            n342 = flat-sequence {
              frame #0 {
                n343 = local write "Sound"(FALSE ("Sound")) -> ()
                n344 = Wait (ms)(milliseconds to wait=u32 3000) -> ()  [unwired: 1 out]
              }
              frame #1 {
                n345 = local write "Sound"(TRUE ("Sound")) -> ()
                n346 = Wait (ms)(milliseconds to wait=u32 50) -> ()  [unwired: 1 out]
              }
              frame #2 {
                n347 = local write "Make sound"(FALSE ("Repeat sound")) -> ()
                n348 = Wait (ms)(milliseconds to wait=u32 10000) -> ()  [unwired: 1 out]
              }
            }
          }
        }
      }
      n349 = while {
        stop <- FALSE stop-if-true
        n350 = flat-sequence {
          frame #0 {
            n351 = while {
              stop <- w404 stop-if-true
              n352 = local read "AIR"() -> (w404:bool)
              n353 = Wait (ms)(milliseconds to wait=u32 50) -> ()  [unwired: 1 out]
            }
          }
          frame #1 {
            n354 = Wait (ms)(milliseconds to wait="Air puff time") -> ()  [unwired: 1 out]
          }
          frame #2 {
            n355 = Wait (ms)(milliseconds to wait=u32 50) -> ()  [unwired: 1 out]
            n356 = local write "AIR"(FALSE ("AIR_L")) -> ()
          }
        }
        n357 = Wait (ms)(milliseconds to wait=u32 50) -> ()  [unwired: 1 out]
      }
      n358 = while "Servo 2 position and LEDs" {
        stop <- FALSE stop-if-true
        n359 = local read "PWM positions"() -> (w471:dbl[])
        n360 = local read "Left"() -> (w472:bool)
        n361 = Wait (ms)(milliseconds to wait=u32 50) -> ()  [unwired: 1 out]
        n362 = case shown="True" w472 {
          tunnel: w471 -> [w478 w484]
          tunnel: [w477 w483] -> w470
          frame False {
            n363 = local read "PWMset1"() -> (w476:dbl[])
            n364 = Index Array(array=w476, index=0) -> (element=w475:dbl)
            n365 = Replace Array Subset(array=w478, new element=w475, index=1) -> (w477:dbl[])
          }
          frame True {
            n366 = local read "PWMset2"() -> (w482:dbl[])
            n367 = Index Array(array=w482, index=0) -> (element=w480:dbl)
            n368 = Replace Array Subset(array=w484, new element=w480, index=1) -> (w483:dbl[])
          }
        }
        n369 = local write "PWM positions"(w470) -> ()
      }
      n370 = while {
        stop <- FALSE stop-if-true
        n371 = flat-sequence {
          frame #0 {
            n372 = while {
              stop <- "Mouse off" stop-if-true
              n373 = Wait (ms)(milliseconds to wait=u32 250) -> ()  [unwired: 1 out]
            }
          }
          frame #1 {
            n374 = for {
              N: 10 -> [_]
              n375 = flat-sequence {
                frame #0 {
                  n376 = local write "LED_L"(TRUE ("LED_L")) -> ()
                  n377 = local write "LED_R"(TRUE ("LED_R")) -> ()
                  n378 = Wait (ms)(milliseconds to wait=u32 1000) -> ()  [unwired: 1 out]
                }
                frame #1 {
                  n379 = local write "LED_R"(FALSE ("LED_R")) -> ()
                  n380 = local write "LED_L"(FALSE ("LED_L")) -> ()
                  n381 = Wait (ms)(milliseconds to wait=u32 1000) -> ()  [unwired: 1 out]
                }
              }
            }
          }
          frame #2 {
            n382 = local write "Mouse off"(FALSE ("Mouse off")) -> ()
          }
        }
      }
      n383 = while {
        stop <- FALSE stop-if-true
        n384 = flat-sequence {
          frame #0 {
            n385 = while {
              stop <- w396 stop-if-true
              n386 = local read "MD_L"() -> (w396:bool)
              n387 = Wait (ms)(milliseconds to wait=u32 50) -> ()  [unwired: 1 out]
            }
          }
          frame #1 {
            n388 = local read "No Milk"() -> (w397:bool)
            n389 = case shown="False" w397 {
              frame False {
                n390 = local read "MD time (ms)"() -> (w398:i32)
                n391 = Wait (ms)(milliseconds to wait=w398) -> ()  [unwired: 1 out]
              }
              frame True {
                n392 = Wait (ms)(milliseconds to wait=u32 50) -> ()  [unwired: 1 out]
              }
            }
          }
          frame #2 {
            w400 = FALSE ("MD_L")
            n393 = Wait (ms)(milliseconds to wait=u32 50) -> ()  [unwired: 1 out]
            n394 = local write "MD_L"(w400) -> ()
            n395 = local write "No Milk"(w400) -> ()
          }
        }
      }
      n396 = while {
        stop <- FALSE stop-if-true
        n397 = flat-sequence {
          frame #0 {
            n398 = while {
              stop <- w388 stop-if-true
              n399 = local read "MD_R"() -> (w388:bool)
              n400 = Wait (ms)(milliseconds to wait=u32 50) -> ()  [unwired: 1 out]
            }
          }
          frame #1 {
            n401 = local read "No Milk"() -> (w389:bool)
            n402 = case shown="False" w389 {
              frame False {
                n403 = local read "MD time (ms)"() -> (w390:i32)
                n404 = Wait (ms)(milliseconds to wait=w390) -> ()  [unwired: 1 out]
              }
              frame True {
                n405 = Wait (ms)(milliseconds to wait=u32 50) -> ()  [unwired: 1 out]
              }
            }
          }
          frame #2 {
            w392 = FALSE ("MD_R")
            n406 = Wait (ms)(milliseconds to wait=u32 50) -> ()  [unwired: 1 out]
            n407 = local write "MD_R"(w392) -> ()
            n408 = local write "No Milk"(w392) -> ()
          }
        }
      }
    }
  }
